vi "Z feedback loop_lateral position readout (SubVI).vi"(4 "PID gains":T1={"proportional gain (Kc)"=0.1, "integral time (Ti, min)"=1.0, "derivative time (Td, min)"=0.0} {"derivative time (Td, min)" format="%.3f"; "integral time (Ti, min)" format="%.3f"; "proportional gain (Kc)" format="%.3f"}, 5 "Polyfit Coeff.":dbl[](array[numeric]), 6 "set z-position (um)":dbl, 7 "current amp.":dbl) -> (1 "z position of PID target (um)":dbl, 2 "z position after moved (um)":dbl)   [LabVIEW 2014]
uses:
  <vilib>/Analysis/polynomials.llb/Scalar Polynomial Evaluation (DBL).vi
  <vilib>/addons/control/pid/pid.llb/PID (DBL).vi
  <vilib>/addons/control/pid/NI_PID_pid.lvlib
  <vilib>/Analysis/NI_AALPro.lvlib
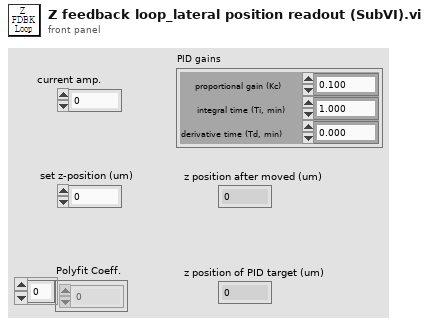
[diagram p1: front panel]
types:
  T1 = cluster{"proportional gain (Kc)":dbl, "integral time (Ti, min)":dbl, "derivative time (Td, min)":dbl}
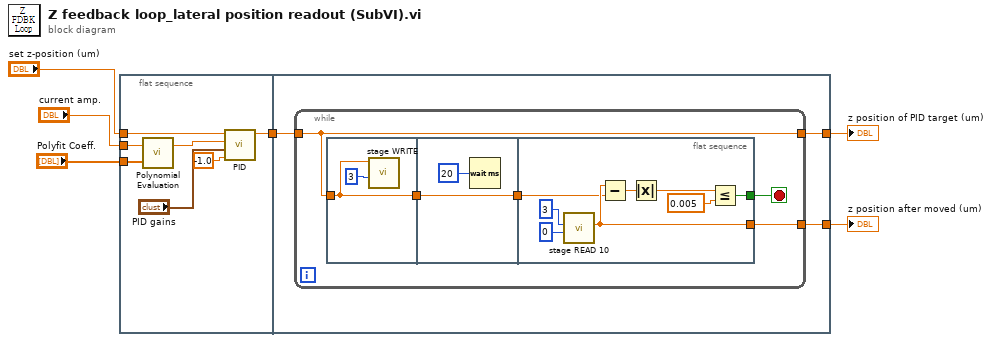
[diagram p0: block diagram]
diagram:
  n1 = flat-sequence {
    tunnel: "set z-position (um)" -> [w13]
    tunnel: "Polyfit Coeff." -> [w12]
    tunnel: "current amp." -> [w11]
    tunnel: [w8] -> w3
    tunnel: w3 -> [w16]
    tunnel: [w15] -> w2
    tunnel: [w14] -> w1
    frame #0 {
      n2 = call-poly <vilib>:"Polynomial Evaluation.vi"("P(x)"=w12, "a"=w11) -> ("P(a)"=w10:dbl)  [unwired: 1 out]
      n3 = call-poly <vilib>:"PID.vi"("dt (s)"=-1.0, "PID gains"="PID gains", "process variable"=w10, "setpoint"=w13) -> ("output"=w8:dbl)  [unwired: 6 in, 1 out]
    }
    frame #1 {
      n4 = while {
        tunnel: w16 -> [w19]
        tunnel: [w20] -> w15
        tunnel: [w19] -> w14
        stop <- w21 stop-if-true
        n5 = flat-sequence {
          tunnel: w19 -> [w22]
          tunnel: [w22] -> w17
          tunnel: [w24] -> w18
          tunnel: w17 -> [w24]
          tunnel: [w33] -> w20
          tunnel: [w32] -> w21
          tunnel: w18 -> [w26]
          frame #0 {
            n6 = call "stage WRITE.vi"("Axis (X1,Y2,Z3)"=u32 3, "Target Position"=w22) -> ()  [unwired: 10 in]
          }
          frame #1 {
            n7 = Wait (ms)(milliseconds to wait=u32 20) -> ()  [unwired: 1 out]
          }
          frame #2 {
            n8 = call "stage READ 10.vi"("ms between measure\n(default=3)"=u32 0 ("ms between measure\n(default=3)"), "Axis (X1,Y2,Z3)"=u32 3) -> ("Position out"=w33:dbl)  [unwired: 9 in]
            n9 = Subtract(x=w33, y=w26) -> (x-y=w28:dbl)
            n10 = Absolute Value(x=w28) -> (abs(x)=w29:dbl)
            n11 = Less Or Equal?(x=w29, y=0.005) -> (x <= y?=w32:bool)
          }
        }
      }
    }
  }
  "z position after moved (um)" <- w2
  "z position of PID target (um)" <- w1
